vi "SMU_Only4Wire Resistance2.vi"(7 "Current_Level":dbl=2e-05 format="%#_6p", 8 "error in (no error)":errorcluster, 9 "Published Data Id":string, 10 "Pins":string[](array[string]), 11 "Semiconductor Module Context":T1) -> (0 "error Out":errorcluster, 2 "R Array":dbl[](array[numeric]), 3 "Semiconductor Module Context Out":T1)   [LabVIEW 2013]
uses:
  <vilib>/NI_TestStand_SemiconductorModule/NI_TestStand_Semiconductor_Module.lvlibp/PinMap/General/SemiconductorModuleContext.ctl
  <vilib>/NI_TestStand_SemiconductorModule/NI_TestStand_Semiconductor_Module.lvlibp/PinMap/DC Power/PinsToNIDCPowerSessions.vi
  <vilib>/NI_TestStand_SemiconductorModule/NI_TestStand_Semiconductor_Module.lvlibp/PinMap/General/Publish/PublishDataDoubleFunctionalTest.vi
  <vilib>/NI_TestStand_SemiconductorModule/NI_TestStand_Semiconductor_Module.lvlibp
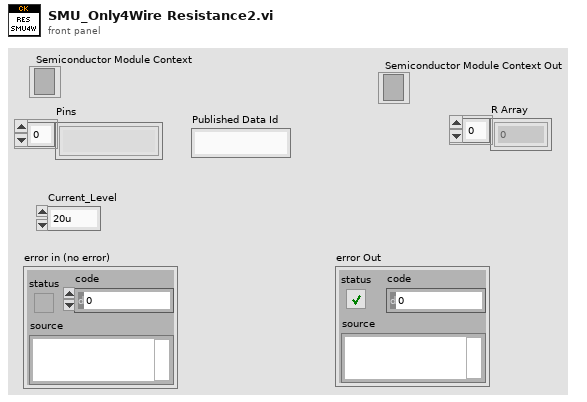
[diagram p1: front panel]
types:
  T1 = typedef "NI_TestStand_Semiconductor_Module.lvlibp/SemiconductorModuleContext.ctl" = refnum<k7>
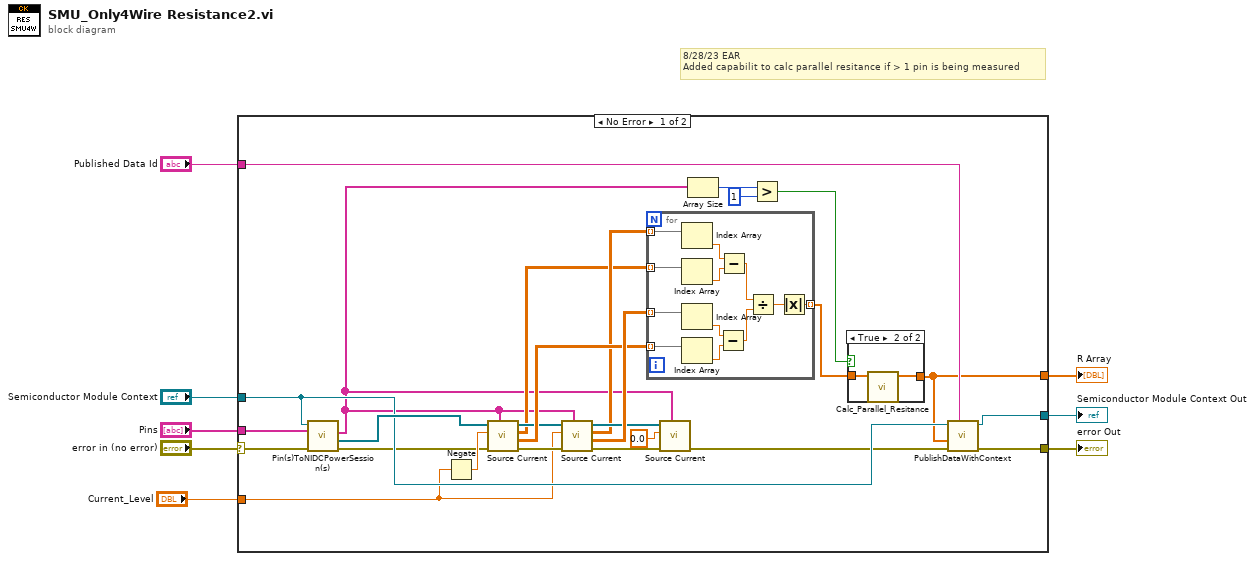
[diagram p0: block diagram]
diagram:
  # "8/28/23 EAR\nAdded capabilit to calc parallel resitance if > 1 pin is being measured"
  n1 = case shown="No Error" "error in (no error)" {
    selector: "error in (no error)" -> [w33 w51]
    tunnel: "Semiconductor Module Context" -> [w21 w50]
    tunnel: "Pins" -> [w22 _]
    tunnel: [w18 w51] -> w5
    tunnel: "Published Data Id" -> [w34 _]
    tunnel: [w27 w50] -> w3
    tunnel: [w11 _] -> w2
    tunnel: "Current_Level" -> [w9 _]
    frame No Error {
      n2 = call-poly <vilib>:"Pin(s)ToNIDCPowerSession(s).vi"("error in (no error)"=w33, "Pins"=w22, "Semiconductor Module Context"=w21) -> ("error out"=w17:errorcluster, "Instrument Sessions"=w30:refnum<k15>[], "Channel Lists"=w15:string[])  [unwired: 4 in, 2 out]
      n3 = Negate(x=w9) -> (-x=w28:dbl)
      n4 = call "Source Current.vi"("Channel Lists"=w15, "error in (no error)"=w17, "current level"=w28, "Instrument Sessions In"=w30) -> ("error out"=w25:errorcluster, "current measurements"=w31:dbl[][], "voltage measurements"=w23:dbl[][], "Instrument Sessions Out"=w24:refnum<k15>[])  [unwired: 4 in]
      n5 = call "Source Current.vi"("Channel Lists"=w15, "error in (no error)"=w25, "current level"=w9, "Instrument Sessions In"=w24) -> ("error out"=w20:errorcluster, "current measurements"=w32:dbl[][], "voltage measurements"=w26:dbl[][], "Instrument Sessions Out"=w29:refnum<k15>[])  [unwired: 4 in]
      n6 = for {
        tunnel: w26 -> [w41] mode=indexing
        tunnel: w32 -> [w49] mode=indexing
        tunnel: [w47] -> w12 mode=indexing
        tunnel: w31 -> [w45] mode=indexing
        tunnel: w23 -> [w38] mode=indexing
        n7 = Index Array(array=w41) -> (element=w40:dbl)  [unwired: 1 in]
        n8 = Index Array(array=w38) -> (element=w39:dbl)  [unwired: 1 in]
        n9 = Index Array(array=w49) -> (element=w42:dbl)  [unwired: 1 in]
        n10 = Index Array(array=w45) -> (element=w44:dbl)  [unwired: 1 in]
        n11 = Subtract(x=w42, y=w44) -> (x-y=w43:dbl)
        n12 = Subtract(x=w40, y=w39) -> (x-y=w46:dbl)
        n13 = Divide(x=w46, y=w43) -> (x/y=w48:dbl)
        n14 = Absolute Value(x=w48) -> (abs(x)=w47:dbl)
      }
      n15 = call "Source Current.vi"("Channel Lists"=w15, "error in (no error)"=w20, "current level"=0.0, "Instrument Sessions In"=w29) -> ("error out"=w19:errorcluster)  [unwired: 4 in, 3 out]
      n16 = Array Size(array=w15) -> (size(s)=w14:i32)
      n17 = Greater?(x=w14, y=1) -> (0:w10:bool)
      n18 = case shown="True" w10 {
        tunnel: w12 -> [w35 w37]
        tunnel: [w35 w36] -> w11
        frame False {
        }
        frame True {
          n19 = call "Calc_Parallel_Resitance.vi"("Resitance_Per Site"=w37) -> ("Parralel_Resistance"=w36:dbl[])  [unwired: 10 in]
        }
      }
      n20 = call-poly <vilib>:"PublishDataWithContext.vi"("Published Data Id"=w34, "error in (no error)"=w19, "Data In"=w11, "Semiconductor Module Context"=w21) -> ("error out"=w18:errorcluster, "Semiconductor Module Context Out"=w27:T1)  [unwired: 6 in]
    }
    frame Error {
    }
  }
  "error Out" <- w5
  "Semiconductor Module Context Out" <- w3
  "R Array" <- w2
